vi "Initialize.vi"(8 "error in (no error)":errorcluster, 9 "Serial Configuration":T1={"Baud Rate"=9600, "Parity"=0, "Stop Bits"=10, "Flow Control"=2} {"Flow Control" items=["None", "XON/XOFF", "RTS/CTS", "XON/XOFF & RTS/CTS", "DTR/DSR", "XON/XOFF & DTR/DSR"]; "Stop Bits" items=["1.0"=10, "1.5"=15, "2.0"=20]; "Parity" items=["None", "Odd", "Even", "Mark", "Space"]; "Baud Rate" items=["300"=300, "600"=600, "1200"=1200, "2400"=2400, "4800"=4800, "9600"=9600, "19200"=19200]}, 11 "Tektronic in":refnum<class "Tektronic.lvclass">) -> (0 "error out":errorcluster, 3 "Tektronic out":refnum<class "Tektronic.lvclass">)   [LabVIEW 2020, in "Controlador.lvlib" / "Tektronic.lvclass"]
uses:
  Tektronic.lvclass
  C:/Users/scrap/Fork/Modulo_Cloneable_DQMH/Libraries/Controlador/Class/Osciloscope/Osciloscope.lvclass
  Osciloscope/Osciloscope.lvclass/Osciloscope.ctl
  Osciloscope/Read COM.vi
  <instrlib>/Tektronix TDS 200 1000 2000 Series/Tektronix TDS 200 1000 2000 Series.lvlib
  Osciloscope/Osciloscope.lvclass
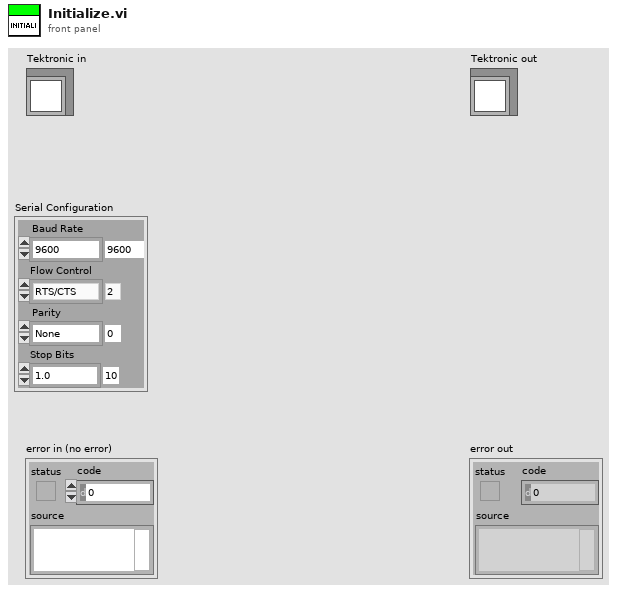
[diagram p1: front panel]
types:
  T1 = cluster{"Baud Rate":u32, "Parity":u16, "Stop Bits":u16, "Flow Control":u16}
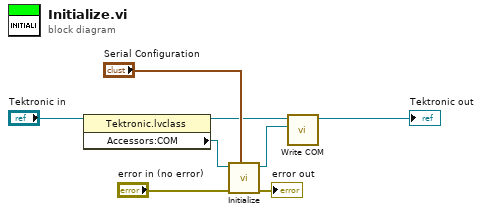
[diagram p0: block diagram]
diagram:
  n1 = property class="Tektronic.lvclass"(reference="Tektronic in") -> (reference out=w3:refnum<class "Tektronic.lvclass">, "Accessors:COM"=w5:refnum<visa-resource-name>)  [unwired: 1 in, 1 out]
  n2 = call <instrlib>:"Initialize.vi"("Serial Configuration"="Serial Configuration", "error in (no error)"="error in (no error)", "VISA resource name"=w5) -> ("error out"=→"error out":errorcluster, "VISA resource name out"=w1:refnum<visa-resource-name>)  [unwired: 7 in]
  n3 = call "Write COM.vi"("COM"=w1, "Osciloscope in"=w3) -> ("Osciloscope out"=→"Tektronic out":refnum<class "Tektronic.lvclass">)  [unwired: 8 in, 1 out]
